vi "生成报表.vi"(11 "缓存数据路径":path=path "C:/Users/Administrator/Desktop/35点监测报警信息报表模板 - 副本.doc") -> ()   [LabVIEW 2017]
uses:
  <vilib>/event_ctls.llb/eventvkey.ctl
  <vilib>/Utility/NIReport.llb/HTML Report Image Alignment.ctl
  <vilib>/Utility/NIReport.llb/Append Report Text (str wrap).vi
  <vilib>/Utility/NIReport.llb/NI_report.lvclass
  <vilib>/Utility/NIReport.llb/NI_ReportGenerationCore.lvlib
panel:
  out "数值":string
  in  "删除文件":bool
  in  "保存":bool
  out "路径显示":path=path "C:/Users/Administrator/Desktop/35点监测报警信息报表模板 - 副本.doc"
  in  "取消":bool
  out "报警等级":string
  in  "生成报表":bool
  out "报警分析":i32(listbox)
  in  "结论":string caption="结论（可编辑）"
  in  "附加信息":string caption="附加信息（可编辑）"
  out "探头信息":string
  out "探头编号":string
  out "实时曲线":cluster{"X":timestamp[], "Y":dbl[]}[](graph)
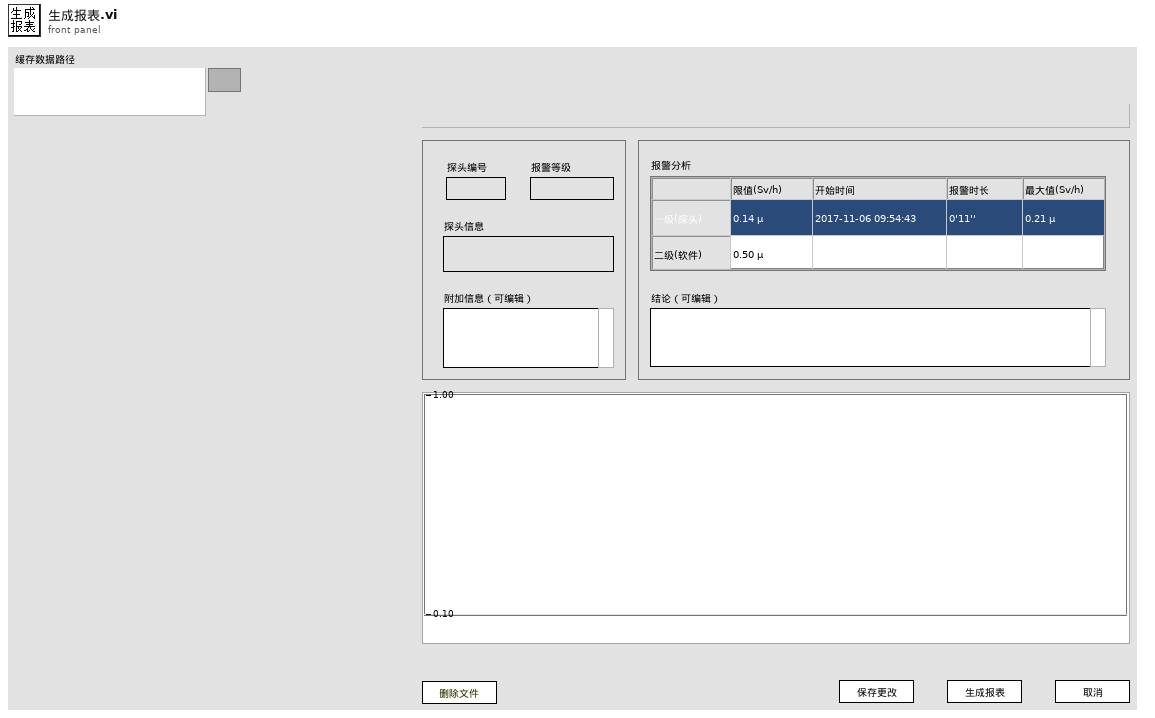
[diagram p1: front panel]
types:
  T1 = enum32{"Invalid", "Standard", "Closed", "Hidden", "Minimized", "Maximized"}
  T2 = typedef "eventvkey.ctl" = enum16{"ASCII", "Enter", "Return", "Shift", "Ctrl", "Alt", "Cmd", "Opt", "Caps", "NumLock", "Clear", "Break", "Up", "Down", "Left", "Right", "Insert", "Delete", "Home", "End", "PageUp", "PageDown", "Escape", "Help", "Pause", "ScrollLock", "F1", "F2", "F3", "F4", "F5", "F6", "F7", "F8", "F9", "F10", "F11", "F12", "F13", "F14", "F15", "F16", "F17", "F18", "F19", "F20", "F21", "F22", "F23", "F24", "Play", "VolumeUp", "VolumeDown", "Mute", "Two Byte Char"}
  T3 = cluster{"position (excel)":cluster{"row":i32, "column":i32}, "name (excel)":string, "bookmark (word)":string}
  T4 = enum16{"Standard Report", "HTML", "Word", "Excel"}
  T5 = enum16{"maximized", "minimized", "normal", "no change"}
  T6 = typedef "NI_ReportGenerationCore.lvlib/HTML Report Image Alignment.ctl" = enum16{"(default)", "LEFT", "RIGHT", "TOP", "TEXTTOP", "MIDDLE", "ABSMIDDLE", "BASELINE", "BOTTOM", "ABSBOTTOM"}
  T7 = cluster{"实时曲线":cluster{"X":timestamp[], "Y":dbl[]}[], "书签-键-值":string[][]}
  T8 = typedef "LVPoint32TypeDef.ctl" = cluster{"Horizontal":i32, "Vertical":i32}
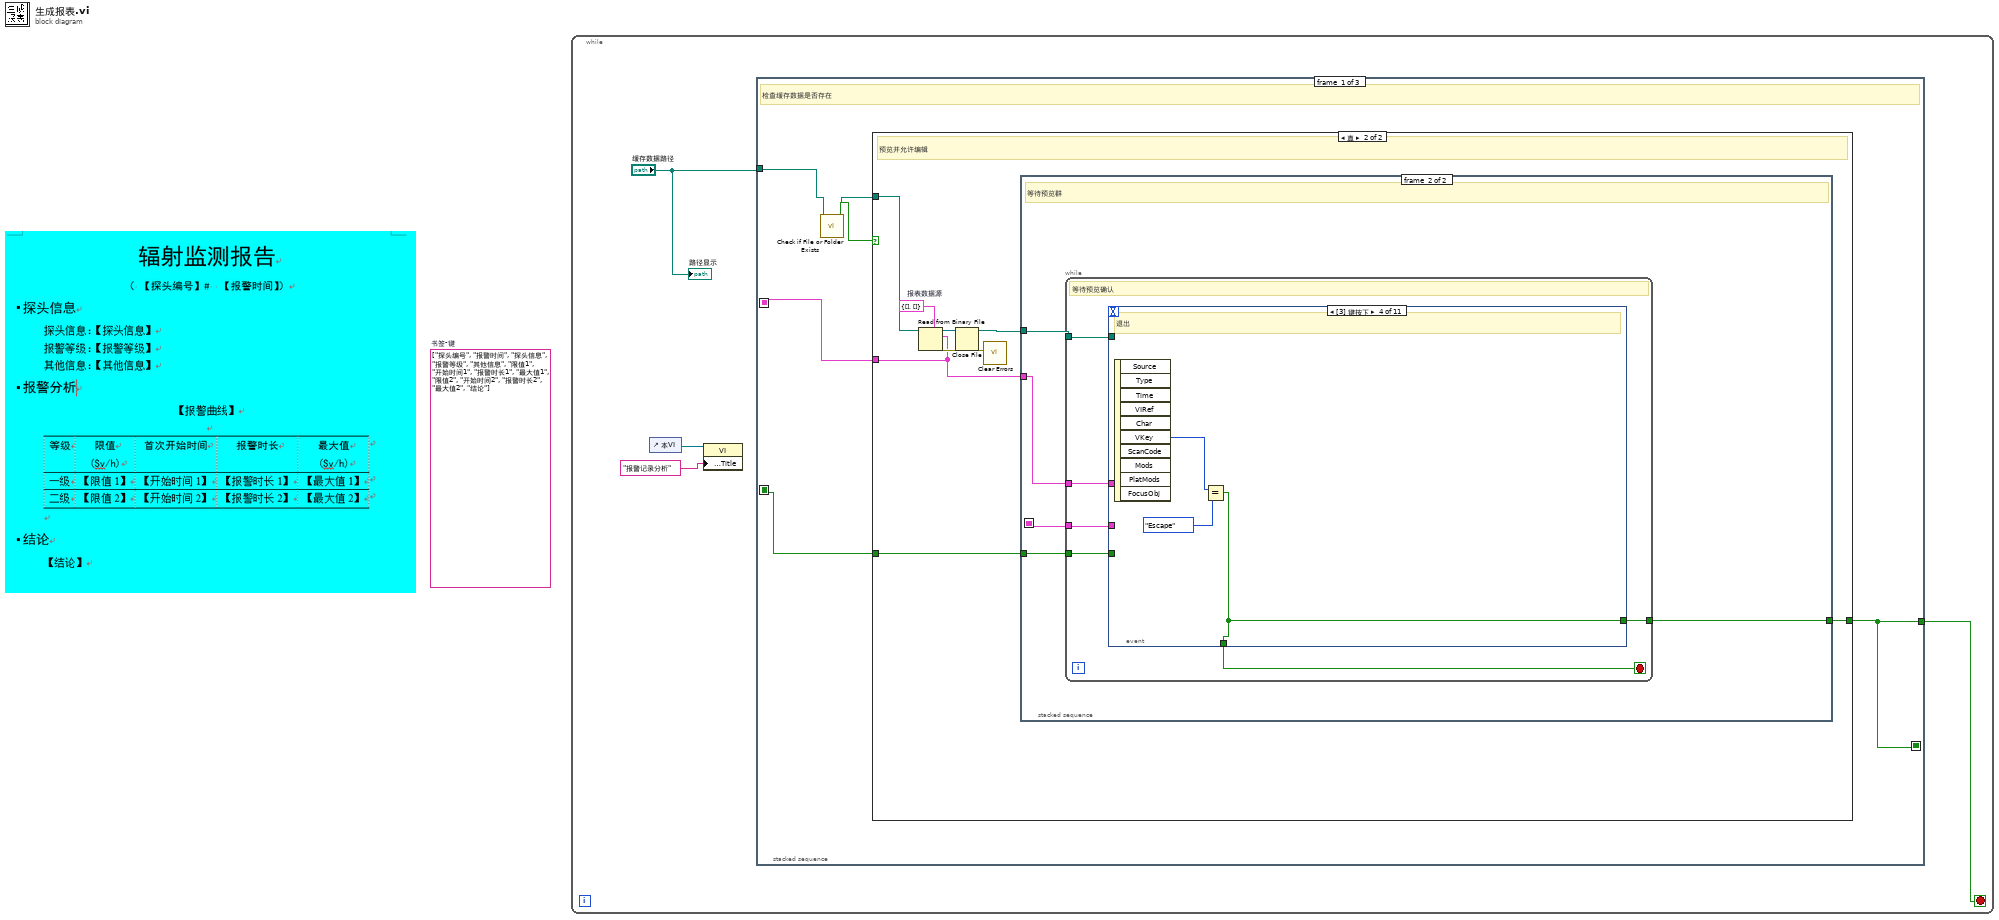
[diagram p0: block diagram]
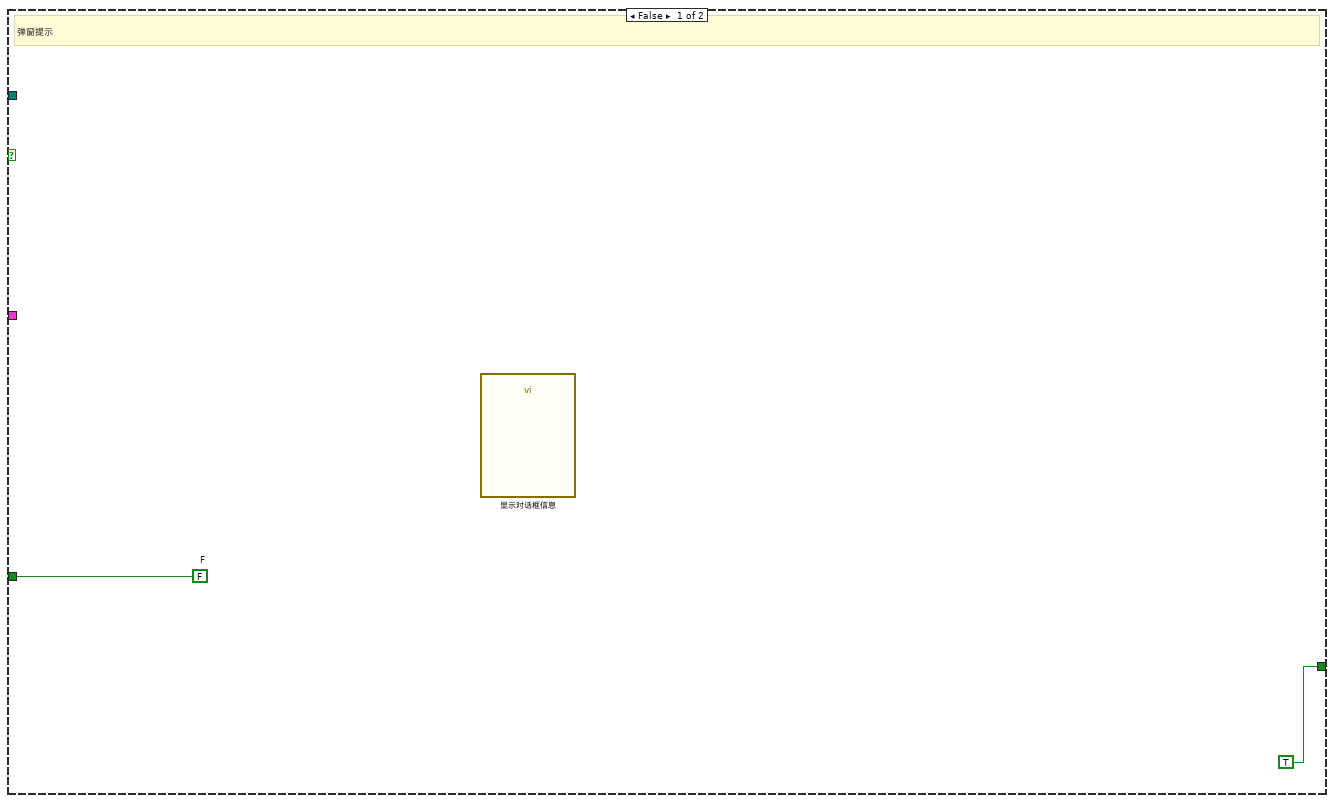
[diagram p2: hidden frame]
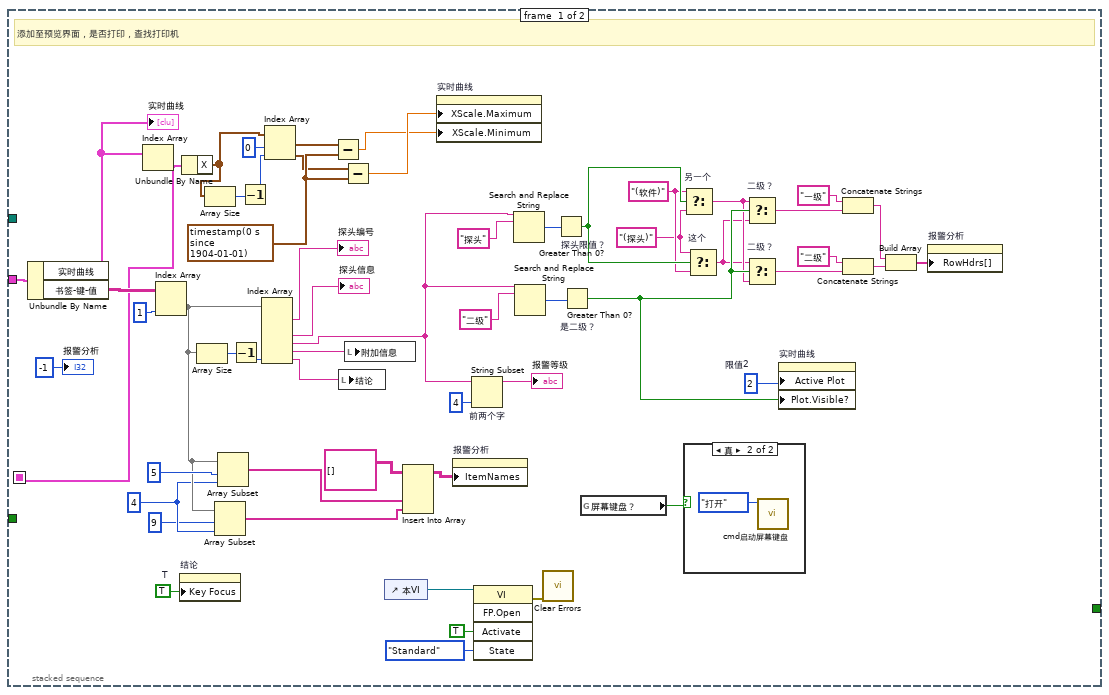
[diagram p3: hidden frame]
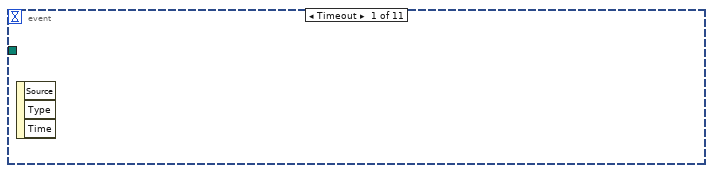
[diagram p5: hidden frame]
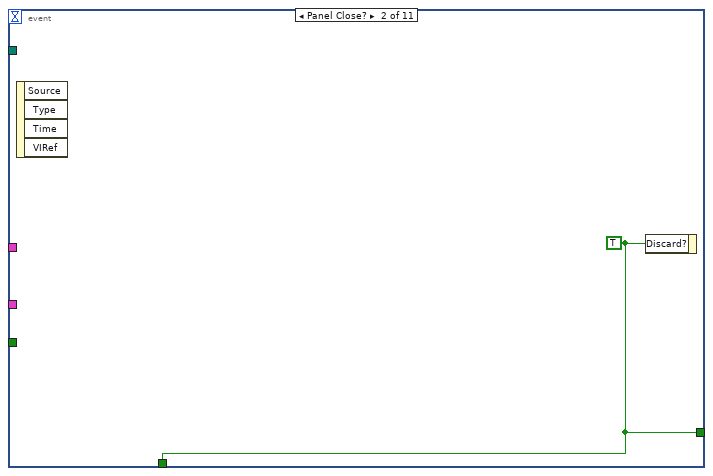
[diagram p6: hidden frame]
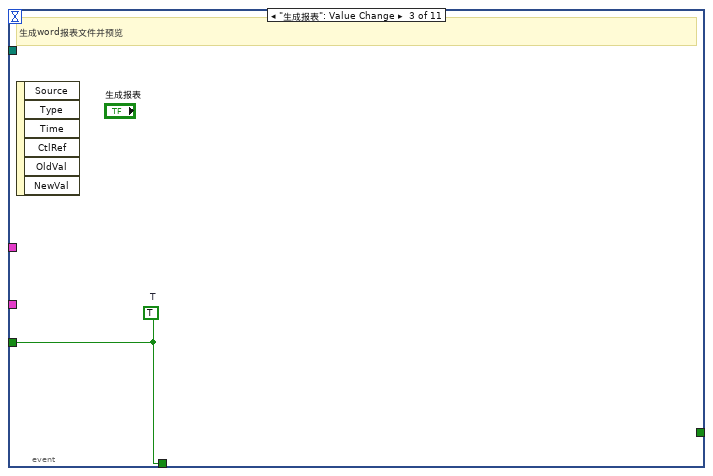
[diagram p7: hidden frame]
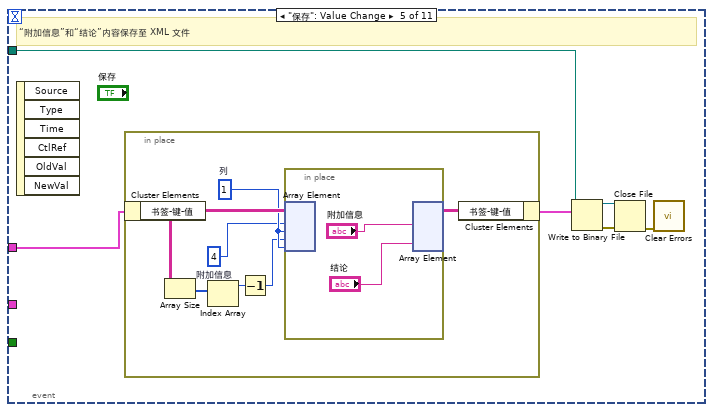
[diagram p8: hidden frame]
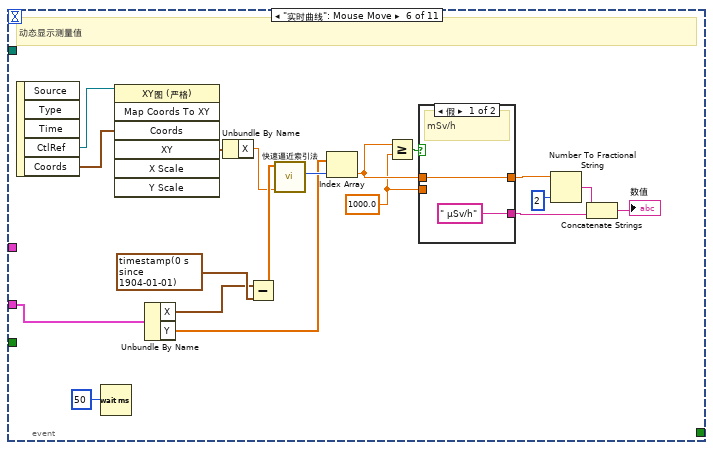
[diagram p9: hidden frame]
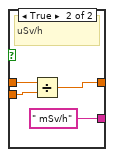
[diagram p10: hidden frame]
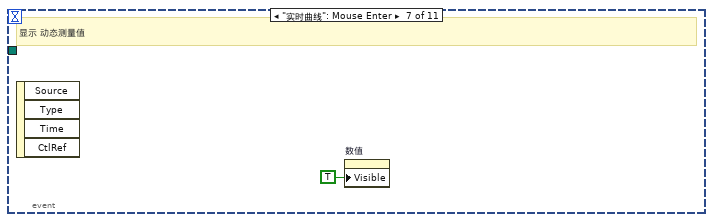
[diagram p11: hidden frame]
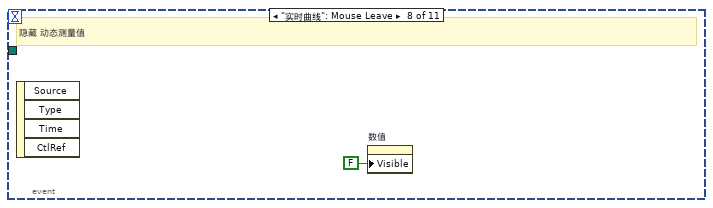
[diagram p12: hidden frame]
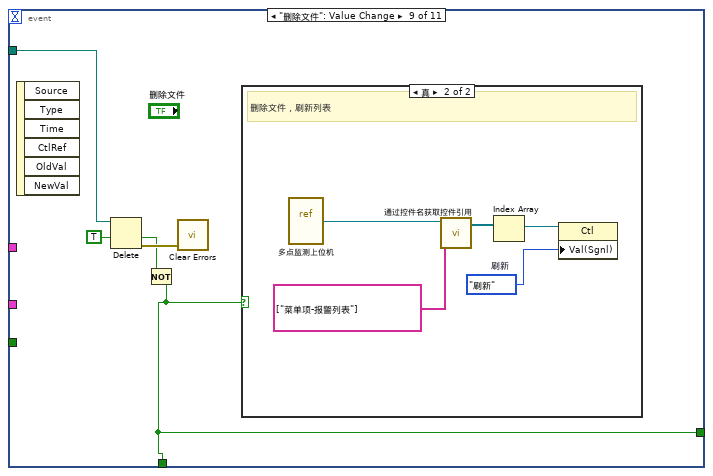
[diagram p13: hidden frame]
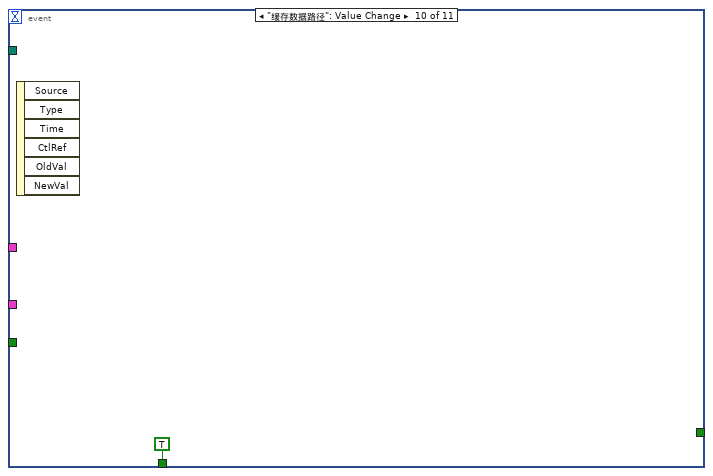
[diagram p15: hidden frame]
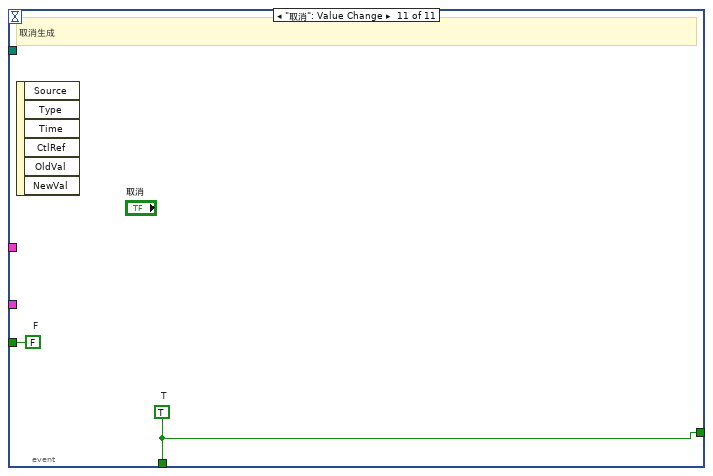
[diagram p16: hidden frame]
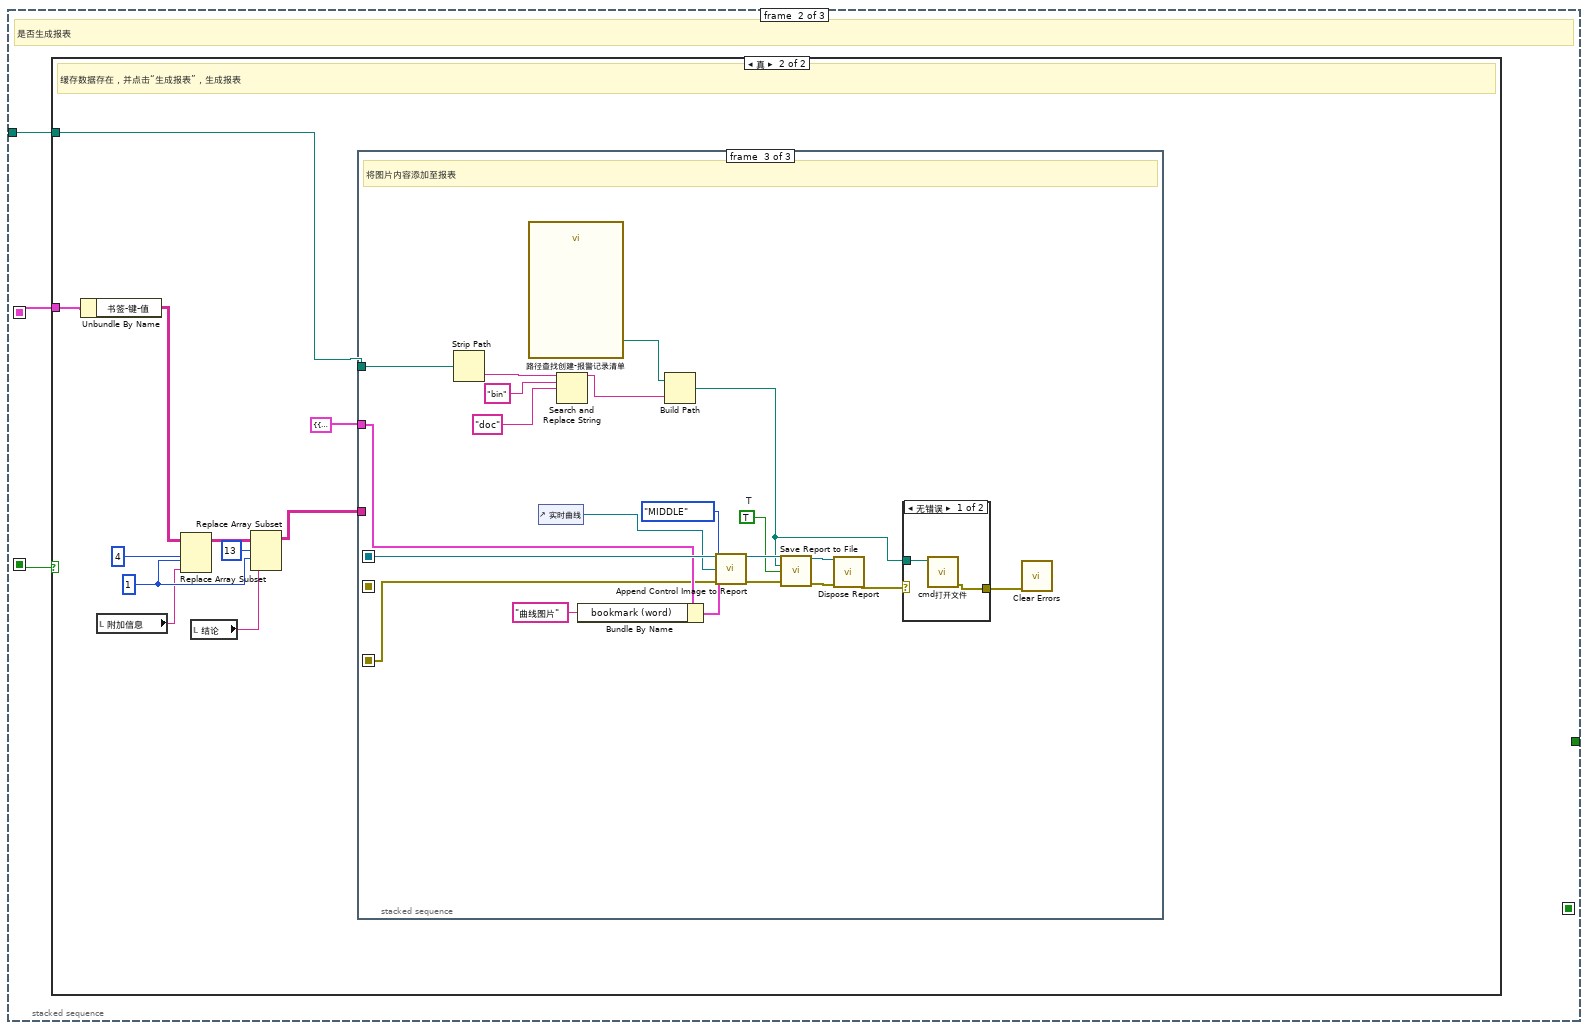
[diagram p17: hidden frame]
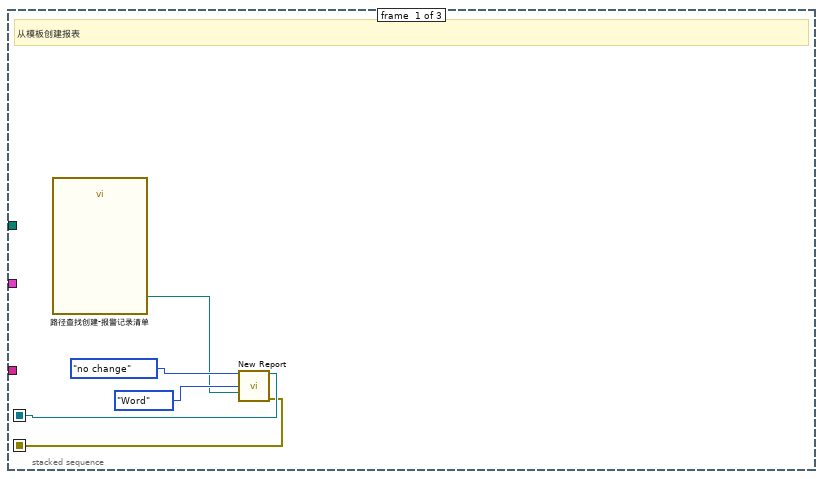
[diagram p19: hidden frame]
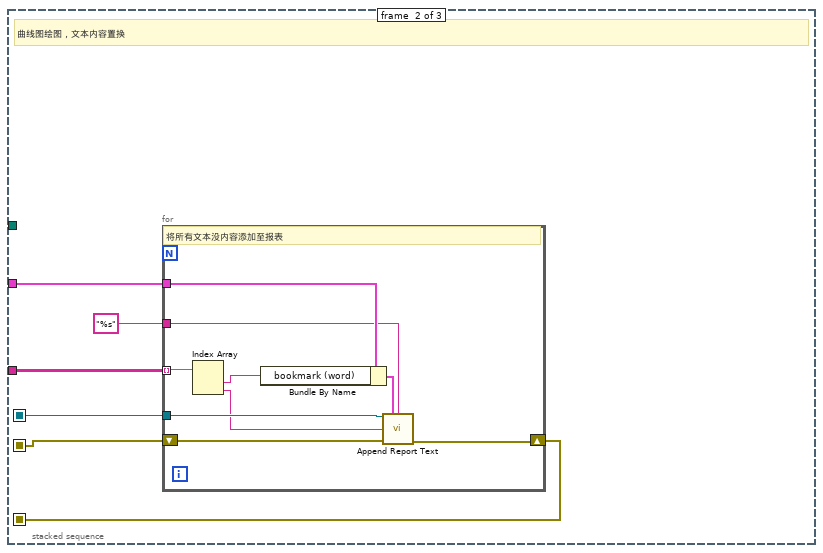
[diagram p20: hidden frame]
diagram:
  (unwired) string[] ["探头编号", "报警时间", "探头信息", "报警等级", "其他信息", "限值1", "开始时间1", "报警时长1", "最大值1", "限值2", "开始时间2", "报警时长2", "最大值2", "结论"]  # 书签-键
  n1 = while {
    stop <- w1 stop-if-true
    n2 = control-ref of="本VI"() -> (w2:refnum<vi>)
    n3 = property class="VI"(reference=w2, "Front Panel.Title"="报警记录分析" ("前面板窗口:标题")) -> ()  [unwired: 1 in, 2 out]
    n4 = stacked-sequence {
      seq-local: [w9 _ _] -> [_ w152 _]
      seq-local: [w10 _ _] -> [_ w151 _]
      seq-local: [w8 _ _] -> [_ _ w208]
      tunnel: "缓存数据路径" -> [w7 w150 _]
      tunnel: [w8 _ _] -> w1
      frame #0 {
        # "检查缓存数据是否存在"
        n5 = call <vilib>:"Check if File or Folder Exists.vi"("path"=w7) -> ("file or folder exists?"=w6:bool, "dup path"=w5:path)  [unwired: 8 in, 1 out]
        n6 = case shown="真" w6 {
          tunnel: [_ w14] -> w10
          tunnel: [w12 w21] -> w9
          tunnel: w5 -> [_ w16]
          tunnel: [TRUE ("确定") w20] -> w8
          frame False {
            w12 = FALSE  # F
            # "弹窗提示"
            n7 = call "显示对话框信息"() -> ()  [unwired: 10 in, 2 out]
          }
          frame True {
            w17 = T7 {"实时曲线"=[], "书签-键-值"=[]}  # 报表数据源
            # "预览并允许编辑"
            n8 = Read from Binary File(5:w17, 11:w16) -> (0:w18:errorcluster, 2:w14:T7, 3:w19:refnum<file>)  [unwired: 4 in, 1 out]
            n9 = Close File(refnum=w19, error in=w18) -> (path=w15:path, error out=w13:errorcluster)
            n10 = call <vilib>:"Clear Errors.vi"("error in (no error)"=w13) -> ()  [unwired: 5 in, 2 out]
            n11 = stacked-sequence {
              seq-local: [w43 _] -> [_ w79]
              tunnel: w14 -> [w77 w82]
              tunnel: [_ w83] -> w21
              tunnel: w15 -> [_ w81]
              tunnel: [_ w80] -> w20
              frame #0 {
                w33 = "(软件)" ("y")
                w29 = "(探头)" ("y")
                w48 = timestamp(0 s since 1904-01-01) ("seconds since 1Jan1904")
                w55 = u32 2  # 限值2
                w60 = TRUE  # T
                w67 = 4 ("索引")
                # "添加至预览界面，是否打印，查找打印机"
                n12 = Unbundle By Name(w77) -> ("实时曲线"=w54:cluster{"X":timestamp[], "Y":dbl[]}[], "书签-键-值"=w76:string[][])
                "实时曲线" <- w54
                n13 = Index Array(array=w54) -> (element=w43:cluster{"X":timestamp[], "Y":dbl[]})  [unwired: 1 in]
                n14 = Index Array(array=w76, index (col)=1 ("禁用的索引 (列)")) -> (element=w68:string[])  [unwired: 1 in]
                n15 = property on="结论" class="Str"("Key Focus"=w60) -> ()  [unwired: 2 in, 2 out]
                n16 = Unbundle By Name(w43) -> ("X"=w50:timestamp[])
                n17 = Array Size(array=w68) -> (size(s)=w71:i32)
                n18 = Array Size(array=w50) -> (size(s)=w53:i32)
                n19 = Array Subset(array=w68, index=9 ("索引"), length=w67) -> (w63:string[])
                n20 = Array Subset(array=w68, index=5 ("索引"), length=w67) -> (w65:string[])
                n21 = Decrement(x=w71) -> (x-1=w70:i32)
                n22 = Decrement(x=w53) -> (x-1=w52:i32)
                n23 = Index Array(array=w68, index #6=w70) -> (element #1=→"探头编号":string, element #3=→"探头信息":string, element #4=w39:string, element #5=w72:string, element #6=w61:string)  [unwired: 5 in, 1 out]
                n24 = Index Array(array=w50, index #1=0 ("索引"), index #2=w52) -> (element #1=w49:timestamp, element #2=w47:timestamp)
                n25 = Subtract(x=w49, y=w48) -> (x-y=w45:dbl)
                n26 = local write "结论"(w61) -> ()
                n27 = Subtract(x=w47, y=w48) -> (x-y=w46:dbl)
                n28 = local write "附加信息"(w72) -> ()
                n29 = control-ref of="本VI"() -> (w59:refnum<vi>)
                n30 = Insert Into Array(array=string[][] [] ("数组"), new element #1=w65, new element #2=w63) -> (w62:string[][])  [unwired: 2 in]
                n31 = property on="实时曲线" class="XYGraph (严格)"("XScale.Maximum"=w46, "XScale.Minimum"=w45) -> ()  [unwired: 2 in, 2 out]
                n32 = property on="报警分析" class="MCListbox (严格)"("ItemNames"=w62) -> ()  [unwired: 2 in, 2 out]
                n33 = String Subset "前两个字"(string=w39, length (rest)=4 ("长度（剩余）")) -> (substring=→"报警等级":string)  [unwired: 1 in]
                n34 = invoke class="VI" method="FP.Open"(reference=w59, "Activate"=TRUE ("激活？"), "State"=T1."Standard" ("状态")) -> (error out=w56:errorcluster)  [unwired: 2 in, 4 out]
                n35 = Search and Replace String(input string=w39, search string="探头" ("y")) -> (number of replacements=w37:i32)  [unwired: 6 in, 3 out]
                n36 = Search and Replace String(input string=w39, search string="二级" ("y")) -> (number of replacements=w40:i32)  [unwired: 6 in, 3 out]
                n37 = call <vilib>:"Clear Errors.vi"("error in (no error)"=w56) -> ()  [unwired: 5 in, 2 out]
                n38 = Greater Than 0? "探头限值？"(x=w37) -> (x > 0?=w34:bool)
                n39 = Greater Than 0? "是二级？"(x=w40) -> (x > 0?=w31:bool)
                n40 = global read "全局变量-35点监测.vi" "屏幕键盘？"() -> (w42:bool)
                n41 = Select "另一个"(t=w33, s=w34, f=w29) -> (s? t:f=w30:string)
                n42 = case shown="真" w42 {
                  frame False {
                  }
                  frame True {
                    n43 = call "cmd启动屏幕键盘.vi"("软键盘开关"=enum16{"关闭", "打开"}."打开") -> ()  [unwired: 9 in, 2 out]
                  }
                }
                n44 = Select "这个"(t=w29, s=w34, f=w33) -> (s? t:f=w22:string)
                n45 = Select "二级？"(t=w30, s=w31, f=w22) -> (s? t:f=w25:string)
                n46 = Select "二级？"(t=w22, s=w31, f=w30) -> (s? t:f=w32:string)
                n47 = property on="实时曲线" class="XYGraph (严格)"("Active Plot"=w55, "Plot.Visible?"=w31) -> ()  [unwired: 2 in, 2 out]
                n48 = Concatenate Strings("一级" ("y"), w25) -> (w28:string)
                n49 = Concatenate Strings("二级" ("y"), w32) -> (w27:string)
                n50 = Build Array(w28, w27) -> (w26:string[])
                n51 = property on="报警分析" class="多列列表框 (严格)"("RowHdrs[]"=w26) -> ()  [unwired: 2 in, 2 out]
                "报警分析" <- -1 ("报警分析")
              }
              frame #1 {
                # "等待预览群"
                n52 = while {
                  tunnel: [w88] -> w83
                  tunnel: w82 -> [w87]
                  tunnel: w81 -> [w86]
                  tunnel: [w85] -> w80
                  tunnel: w79 -> [w84]
                  stop <- w89 stop-if-true
                  # "等待预览确认"
                  n53 = event shown="[3] 键按下" {
                    selector: _ -> [_ _ _ _ _ _ _ _ _ _ _]
                    dyn-events: _ -> [_ _ _ _ _ _ _ _ _ _ _]
                    timeout: _ -> [_ _ _ _ _ _ _ _ _ _ _]
                    tunnel: [_ w90 w91 w92 _ _ _ _ w137 TRUE ("T") w148] -> w89
                    tunnel: [_ _ w91 _ _ _ _ _ _ _ w149] -> w88
                    tunnel: w87 -> [_ _ _ _ w100 _ _ _ _ _ _]
                    tunnel: w86 -> [_ _ _ _ w95 _ _ _ w141 _ _]
                    tunnel: [_ w90 _ w92 _ _ _ _ w137 _ w148] -> w85
                    tunnel: w84 -> [_ _ _ _ _ w110 _ _ _ _ _]
                    event Timeout {
                      n54 = event-data() -> ()  [unwired: 1 in, 3 out]
                    }
                    event Panel Close? {
                      w90 = TRUE ("放弃？")
                      n55 = event-data() -> ()  [unwired: 1 in, 4 out]
                      n56 = event-data("Discard?"=w90) -> ()  [unwired: 1 in, 1 out]
                    }
                    event "生成报表": Value Change {
                      w91 = TRUE  # T
                      # "生成word报表文件并预览"
                      n57 = event-data() -> ()  [unwired: 1 in, 6 out]
                    }
                    event Key Down {
                      # "退出"
                      n58 = event-data() -> ("VKey"=w94:T2)  [unwired: 1 in, 9 out]
                      n59 = Equal?(x=w94, y=eventvkey."Escape") -> (x = y?=w92:bool)
                    }
                    event "保存": Value Change {
                      # "“附加信息”和“结论”内容保存至 XML 文件"
                      n60 = event-data() -> ()  [unwired: 1 in, 6 out]
                      n61 = in-place {
                        w103 = 1  # 列
                        w102 = 4  # 附加信息
                        n62 = in-place-cluster #1(w100) -> ("书签-键-值"=w107:string[][])
                        n63 = Array Size(array=w107) -> (size(s)=w106:i32[])
                        n64 = Index Array(array=w106) -> (element=w105:i32)  [unwired: 1 in]
                        n65 = Decrement(x=w105) -> (x-1=w101:i32)
                        n66 = in-place {
                          n67 = in-place-array #2(w107, w102, w103, w101, w103) -> ()  [unwired: 2 out]
                          n68 = in-place-array #2("附加信息", "结论") -> (w104:string[][])  [unwired: 4 out]
                        }
                        n69 = in-place-cluster #1("书签-键-值"=w104) -> (w96:T7)
                      }
                      n70 = Write to Binary File(file (use dialog)=w95, data=w96) -> (refnum out=w98:refnum<file>, error out=w99:errorcluster)  [unwired: 4 in, 1 out]
                      n71 = Close File(refnum=w98, error in=w99) -> (error out=w97:errorcluster)  [unwired: 1 out]
                      n72 = call <vilib>:"Clear Errors.vi"("error in (no error)"=w97) -> ()  [unwired: 5 in, 2 out]
                    }
                    event "实时曲线": Mouse Move {
                      w116 = 1000.0 ("y")
                      # "动态显示测量值"
                      n73 = event-data() -> ("CtlRef"=w111:refnum<vi>, "Coords"=w112:T8)  [unwired: 1 in, 3 out]
                      n74 = Wait (ms)(milliseconds to wait=u32 50 ("等待时间（毫秒）")) -> ()  [unwired: 1 out]
                      n75 = invoke on="调用节点" class="XY图 (严格)" method="Map Coords To XY"(reference=w111, "Coords"=w112) -> ("XY"=w114:cluster{"X":dbl, "Y":dbl})  [unwired: 5 in, 6 out]
                      n76 = Unbundle By Name(w110) -> ("X"=w123:timestamp[], "Y"=w126:dbl[])
                      n77 = Unbundle By Name(w114) -> ("X"=w122:dbl)
                      n78 = Subtract(x=w123, y=timestamp(0 s since 1904-01-01)) -> (x-y=w125:dbl[])
                      n79 = call "快速逼近索引法.vi"("数值"=w122, "数组"=w125) -> ("最近索引"=w127:i32)  [unwired: 9 in]
                      n80 = Index Array(array=w126, index=w127) -> (element=w128:dbl)
                      n81 = Greater Or Equal?(x=w128, y=w116) -> (x >= y?=w115:bool)
                      n82 = case shown="假" w115 {
                        tunnel: w128 -> [w130 w134]
                        tunnel: w116 -> [_ w133]
                        tunnel: [w130 w132] -> w118
                        tunnel: [" μSv/h" " mSv/h"] -> w120
                        frame False {
                          # "mSv/h"
                        }
                        frame True {
                          # "uSv/h"
                          n83 = Divide(x=w134, y=w133) -> (x/y=w132:dbl)
                        }
                      }
                      n84 = Number To Fractional String(number=w118, precision (6)=i16 2 ("精度(6)")) -> (F-format string=w119:string)  [unwired: 2 in]
                      n85 = Concatenate Strings(w119, w120) -> (→"数值":string)
                    }
                    event "实时曲线": Mouse Enter {
                      # "显示 动态测量值"
                      n86 = event-data() -> ()  [unwired: 1 in, 4 out]
                      n87 = property on="数值" class="Str"("Visible"=TRUE ("可见")) -> ()  [unwired: 2 in, 2 out]
                    }
                    event "实时曲线": Mouse Leave {
                      # "隐藏 动态测量值"
                      n88 = event-data() -> ()  [unwired: 1 in, 4 out]
                      n89 = property on="数值" class="Str"("Visible"=FALSE ("可见")) -> ()  [unwired: 2 in, 2 out]
                    }
                    event "删除文件": Value Change {
                      n90 = event-data() -> ()  [unwired: 1 in, 6 out]
                      n91 = Delete(path (use dialog)=w141, confirm (F)=TRUE ("确认(F)")) -> (cancelled=w138:bool, error out=w140:errorcluster)  [unwired: 3 in, 1 out]
                      n92 = Not(x=w138) -> (.not. x?=w137:bool)
                      n93 = call <vilib>:"Clear Errors.vi"("error in (no error)"=w140) -> ()  [unwired: 5 in, 2 out]
                      n94 = case shown="真" w137 {
                        frame False {
                          # "取消删除"
                        }
                        frame True {
                          w142 = enum16{"刷新", "预览并生成报表", "删除记录", "复制选中项至剪贴板"}."刷新"  # 刷新
                          # "删除文件，刷新列表"
                          n95 = vi-ref "多点监测上位机.vi"() -> (w146:refnum<vi>)
                          n96 = call "通过控件名获取控件引用.vi"("控件名数组"=string[] ["菜单项-报警列表"], "VI引用"=w146) -> ("控件引用输出"=w144:refnum<vi>[])  [unwired: 7 in, 2 out]
                          n97 = Index Array(array=w144) -> (element=w143:refnum<vi>)  [unwired: 1 in]
                          n98 = property class="Ctl"(reference=w143, "Val(Sgnl)"=w142) -> ()  [unwired: 1 in, 2 out]
                        }
                      }
                    }
                    event "缓存数据路径": Value Change {
                      n99 = event-data() -> ()  [unwired: 1 in, 6 out]
                    }
                    event "取消": Value Change {
                      w149 = FALSE  # F
                      w148 = TRUE  # T
                      # "取消生成"
                      n100 = event-data() -> ()  [unwired: 1 in, 6 out]
                    }
                  }
                }
              }
            }
          }
        }
      }
      frame #1 {
        # "是否生成报表"
        n101 = case shown="真" w152 {
          tunnel: w151 -> [_ w163]
          tunnel: w150 -> [_ w161]
          frame False {
            # "缓存数据不存在，或点击“取消”"
          }
          frame True {
            w157 = 1 ("禁用的索引 (列)")
            # "缓存数据存在，并点击“生成报表”，生成报表"
            n102 = Unbundle By Name(w163) -> ("书签-键-值"=w160:string[][])
            n103 = local read "附加信息"() -> (w155:string)
            n104 = Replace Array Subset(array=w160, new element=w155, index (row)=4 ("禁用的索引 (行)"), index (col)=w157) -> (w158:string[][])
            n105 = local read "结论"() -> (w154:string)
            n106 = Replace Array Subset(array=w158, new element=w154, index (row)=13 ("禁用的索引 (行)"), index (col)=w157) -> (w153:string[][])
            n107 = stacked-sequence {
              seq-local: [w166 _ _] -> [_ w173 w202]
              seq-local: [_ w169 _] -> [_ _ w188]
              seq-local: [w164 _ _] -> [_ w170 _]
              tunnel: w153 -> [_ w174 _]
              tunnel: T3 {"position (excel)"={"row"=0, "column"=0}, "name (excel)"="", "bookmark (word)"=""} ("MS Office parameters") -> [_ w171 w200]
              tunnel: w161 -> [_ _ w197]
              frame #0 {
                # "从模板创建报表"
                n108 = call "路径查找创建-报警记录清单.vi"() -> ("报表模板"=w165:path)  [unwired: 8 in, 11 out]
                n109 = call <vilib>:"New Report.vi"("window state (normal)"=T5."no change", "report type"=T4."Word", "template (empty)"=w165) -> ("report out"=w166:refnum<class "NI_report.lvclass">, "error out"=w164:errorcluster)  [unwired: 11 in]
              }
              frame #1 {
                # "曲线图绘图，文本内容置换"
                n110 = for {
                  tunnel: w174 -> [w183] mode=indexing
                  tunnel: w171 -> [w182]
                  tunnel: w173 -> [w179]
                  tunnel: "%s" ("format string (%.3f)") -> [w177]
                  shift-right: [w176] -> w169
                  shift-left: w170 -> [w175]
                  # "将所有文本没内容添加至报表"
                  n111 = Index Array(array=w183) -> (element #1=w181:string, element #2=w178:string)  [unwired: 2 in]
                  n112 = Bundle By Name(cluster=w182, "bookmark (word)"=w181) -> (w180:T3)
                  n113 = call-poly <vilib>:"Append Report Text.vi"("report in"=w179, "MS Office parameters"=w180, "format string (%.3f)"=w177, "text"=w178, "error in (no error)"=w175) -> ("error out"=w176:errorcluster)  [unwired: 7 in, 3 out]
                }
              }
              frame #2 {
                w190 = TRUE  # T
                # "将图片内容添加至报表"
                n114 = Strip Path(path=w197) -> (name=w196:string)  [unwired: 1 out]
                n115 = call "路径查找创建-报警记录清单.vi"() -> ("报表文件夹"=w193:path)  [unwired: 8 in, 11 out]
                n116 = control-ref of="实时曲线"() -> (w199:refnum<vi>)
                n117 = Search and Replace String(input string=w196, search string="bin" ("搜索字符串"), replace string="doc" ("搜索字符串")) -> (result string=w192:string)  [unwired: 5 in, 3 out]
                n118 = Bundle By Name(cluster=w200, "bookmark (word)"="曲线图片") -> (w201:T3)
                n119 = Build Path(base path=w193, name or relative path=w192) -> (appended path=w185:path)
                n120 = call-dynamic "Append Control Image to Report.vi"("report in"=w202, "alignment (default)"=HTML_Report_Image_Alignment."MIDDLE", "ctrl reference"=w199, "error in (no error)"=w188, "MS Office parameters"=w201) -> ("report out"=w191:refnum<class "NI_report.lvclass">, "error out"=w189:errorcluster)  [unwired: 7 in, 2 out]
                n121 = call-dynamic "Save Report to File.vi"("report in"=w191, "report file path"=w185, "prompt to replace? (F)"=w190, "error in (no error)"=w189) -> ("report out"=w198:refnum<class "NI_report.lvclass">, "error out"=w187:errorcluster)  [unwired: 10 in]
                n122 = call-dynamic "Dispose Report.vi"("report in"=w198, "error in (no error)"=w187) -> ("error out"=w184:errorcluster)  [unwired: 13 in]
                n123 = case shown="无错误" w184 {
                  selector: w184 -> [_ w207]
                  tunnel: [w206 w207] -> w186
                  tunnel: w185 -> [w205 _]
                  frame No Error {
                    n124 = call "cmd打开文件.vi"("文件路径"=w205) -> ("error out"=w206:errorcluster)  [unwired: 10 in]
                  }
                  frame Error {
                  }
                }
                n125 = call <vilib>:"Clear Errors.vi"("error in (no error)"=w186) -> ()  [unwired: 5 in, 2 out]
              }
            }
          }
        }
      }
      frame #2 {
        # "退出关闭本VI"
        n126 = case shown="真" w208 {
          frame False {
          }
          frame True {
            # "结束程序？"
            n127 = control-ref of="本VI"() -> (w214:refnum<vi>)
            n128 = call "cmd启动屏幕键盘.vi"("软键盘开关"=enum16{"关闭", "打开"}."关闭") -> ("error out"=w209:errorcluster)  [unwired: 9 in, 1 out]
            n129 = invoke class="VI" method="FP.Close"(reference=w214, error in=w209) -> (reference out=w213:refnum<vi>, error out=w212:errorcluster)  [unwired: 1 in, 1 out]
            n130 = invoke class="VI" method="Abort VI"(reference=w213, error in=w212) -> (error out=w211:errorcluster)  [unwired: 1 in, 2 out]
            n131 = call <vilib>:"Clear Errors.vi"("error in (no error)"=w211) -> ()  [unwired: 5 in, 2 out]
          }
        }
      }
    }
    "路径显示" <- "缓存数据路径"
  }
